vi "Choreo_TrajectorySwerve_Samples.vi"(11 "ChoreoTrajectorySwerve":T2) -> (3 "samples":T1[](array[typedef]))   [LabVIEW 2019, in "ChoreoLib.lvlib"]
doc: "Returns the samples of the trajectory.\n \nInputs:\n -- ChoreoTrajectorySwerve - cluster - data cluster for this trajectory \n\nOutputs: \n -- samples - SwerveSample - the samples of the trajectory."
uses:
  ChoreoLib.lvlib
  TypeDef/ChoreoTrajectorySwerve.ctl
  TypeDef/ChoreoSwerveSample.ctl
  TypeDef/ChoreoEventMarker.ctl
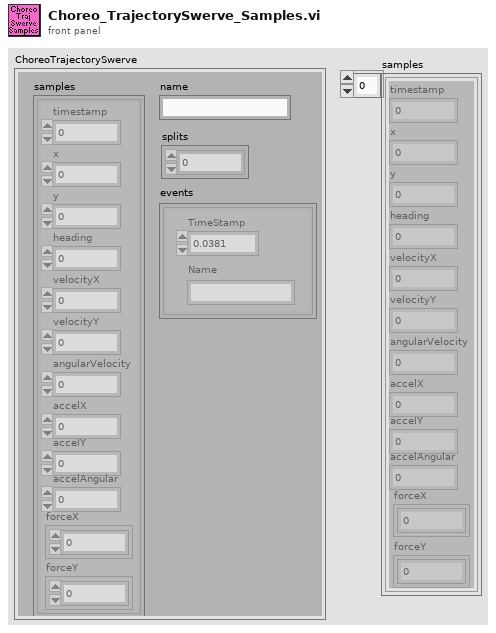
[diagram p1: front panel]
types:
  T1 = typedef "ChoreoLib.lvlib/ChoreoSwerveSample.ctl" = cluster{"timestamp":dbl, "x":dbl, "y":dbl, "heading":dbl, "velocityX":dbl, "velocityY":dbl, "angularVelocity":dbl, "accelX":dbl, "accelY":dbl, "accelAngular":dbl, "forceX":dbl[], "forceY":dbl[]}
  T2 = typedef "ChoreoLib.lvlib/ChoreoTrajectorySwerve.ctl" = cluster{"name":string, "samples":T1[], "splits":i32[], "events":T3[]}
  T3 = typedef "ChoreoLib.lvlib/ChoreoEventMarker.ctl" = cluster{"TimeStamp":dbl, "Name":string}
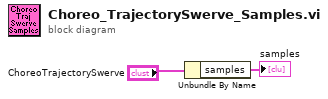
[diagram p0: block diagram]
diagram:
  n1 = Unbundle By Name("ChoreoTrajectorySwerve") -> ("samples"=→"samples":T1[])
